vi "Read TopRef.vi"(8 "error in (no error)":errorcluster, 11 "UIActorTop2 in":refnum<class "UI_Left_Right.lvclass">) -> (0 "error out":errorcluster, 2 "TopRef":T1, 3 "UIActorTop2 out":refnum<class "UI_Left_Right.lvclass">)   [LabVIEW 2021, in "UI_Left_Right.lvclass"]
uses:
  UI_Left_Right.lvclass
  TopRef.ctl
  UI_Left_Right.lvclass/UI_Left_Right.ctl
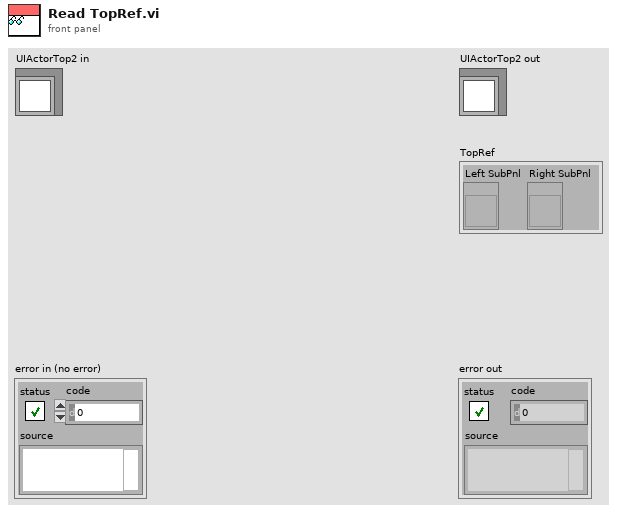
[diagram p1: front panel]
types:
  T1 = typedef "UI_Left_Right.lvclass/TopRef.ctl" = cluster{"Left SubPnl":refnum<vi>, "Right SubPnl":refnum<vi>}
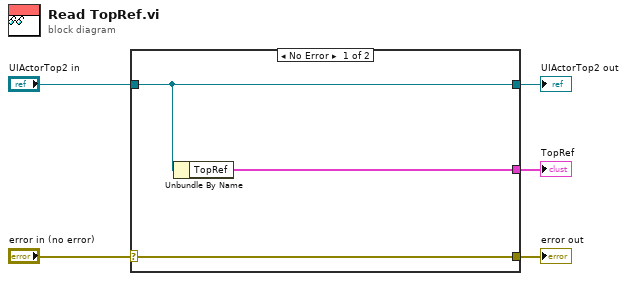
[diagram p0: block diagram]
diagram:
  n1 = case shown="No Error" "error in (no error)" {
    selector: "error in (no error)" -> [w8 w9]
    tunnel: [w8 w9] -> w4
    tunnel: [w7 w10] -> w2
    tunnel: "UIActorTop2 in" -> [w7 w10]
    tunnel: [w6 _] -> w1
    frame No Error {
      n2 = Unbundle By Name(w7) -> ("TopRef"=w6:T1)
    }
    frame Error {
    }
  }
  "error out" <- w4
  "UIActorTop2 out" <- w2
  "TopRef" <- w1
